vi "Warning Incriment.vi"(5 "Numeric 2":i32, 6 "Array 2":i32[](array[numeric]), 7 "Warning Queue In":string, 8 "Warning In":string, 9 "Warning\nOccured In":bool, 10 "Warning Input":i32) -> (0 "Warning Queue Out":string, 1 "Warning Out":string, 2 "Warning\nOccured Out":bool, 3 "Warning Output":i32, 4 "Array 3":i32[](array[numeric]))   [LabVIEW 2013]
panel:
  out "concatenated string":string
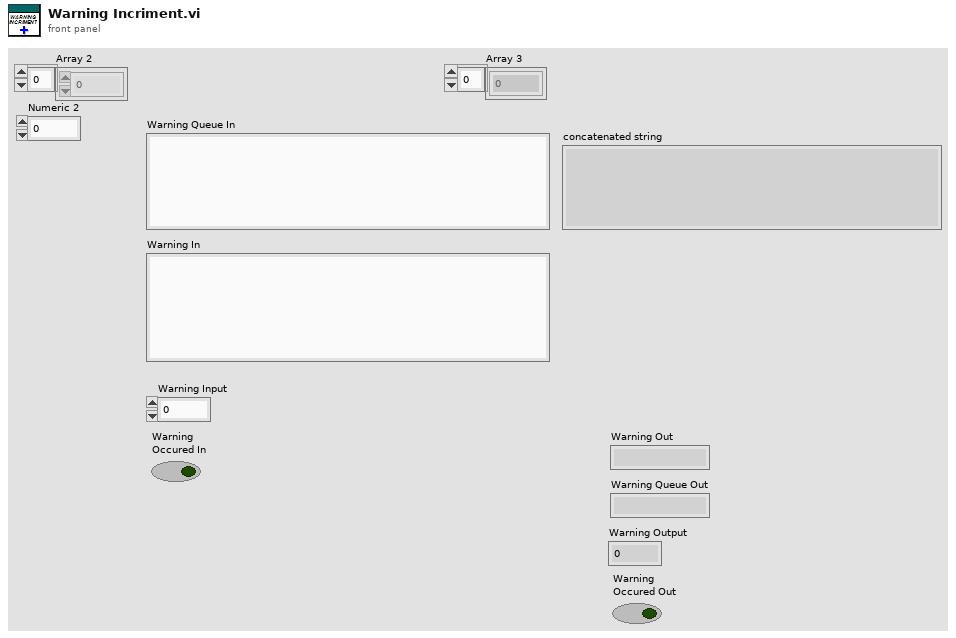
[diagram p1: front panel]
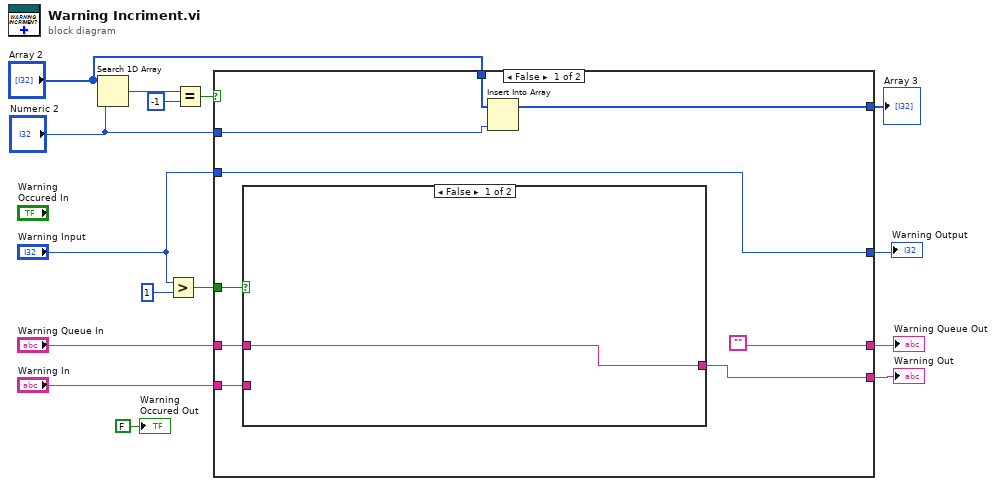
[diagram p0: block diagram]
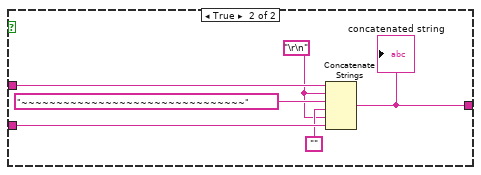
[diagram p2: hidden frame]
diagram:
  n1 = Search 1D Array(1D array="Array 2", element="Numeric 2") -> (index of element=w4:i32)  [unwired: 1 in]
  n2 = Greater?(x="Warning Input", y=1) -> (0:w11:bool)
  n3 = Equal?(x=w4, y=-1) -> (x = y?=w6:bool)
  n4 = case shown="False" w6 {
    tunnel: "Warning Queue In" -> [w24 w34]
    tunnel: "Warning In" -> [w23 w33]
    tunnel: w11 -> [w22 _]
    tunnel: "Warning Input" -> [w21 w35]
    tunnel: [w21 w35] -> w9
    tunnel: ["" w34] -> w8
    tunnel: [w19 w33] -> w7
    tunnel: "Numeric 2" -> [w18 _]
    tunnel: "Array 2" -> [w17 w32]
    tunnel: [w16 w32] -> w1
    frame False {
      n5 = case shown="False" w22 {
        tunnel: w24 -> [w25 w30]
        tunnel: [w25 w31] -> w19
        tunnel: w23 -> [_ w28]
        frame False {
        }
        frame True {
          w26 = "\r\n"
          n6 = Concatenate Strings(w30, w26, "~~~~~~~~~~~~~~~~~~~~~~~~~~~~~~~~" ("string"), "", w26, w28) -> (w31:string)
          "concatenated string" <- w31
        }
      }
      n7 = Insert Into Array(array=w17, new element=w18) -> (w16:i32[])  [unwired: 1 in]
    }
    frame True {
    }
  }
  "Warning Output" <- w9
  "Warning Queue Out" <- w8
  "Warning Out" <- w7
  "Array 3" <- w1
  "Warning\nOccured Out" <- FALSE ("Warning\nIncriment 2")
